vi "DecodeBase64ToImageFile.vi"(8 "error in (no error)":errorcluster, 9 "Base64String":string, 11 "Output FilePath":path) -> (0 "error out":errorcluster, 3 "Output FilePath (FileExtensionAdapted)":path)   [LabVIEW 2020]
doc: "Decode a Base64 Image to a file"
uses:
  <userlib>/_OpenG.lib/file/file.llb/Valid Path - Traditional__ogtk.vi
  <vilib>/Utility/error.llb/Error Cluster From Error Code.vi
  <userlib>/_OpenG.lib/file/file.llb/Convert File Extension (Path)__ogtk.vi
  <vilib>/ErrorRing/Error Ring.xnode
  <userlib>/_OpenG.lib/file/file.llb/openg_file.lvlib
  <vilib>/JDP Science/JDP Science Common Utilities/Base64/Base64 Support.lvlib
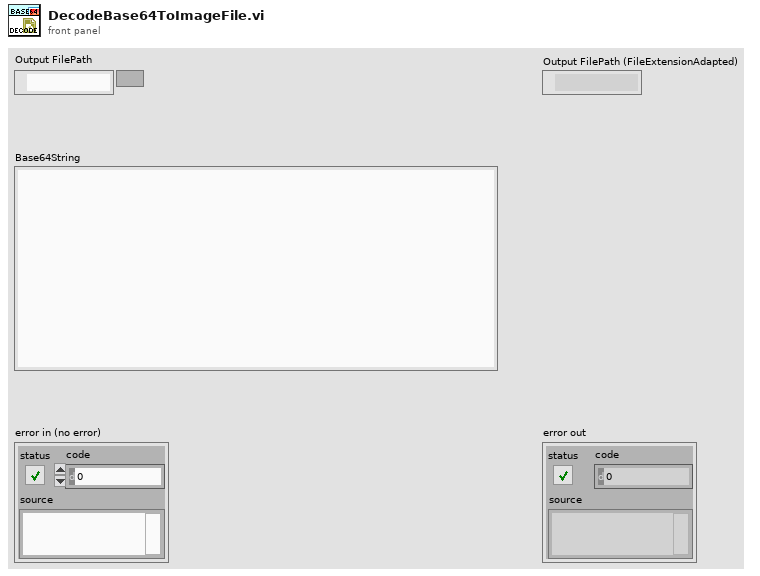
[diagram p1: front panel]
types:
  T1 = enum16{"open", "replace", "create", "open or create", "replace or create", "replace or create with confirmation"}
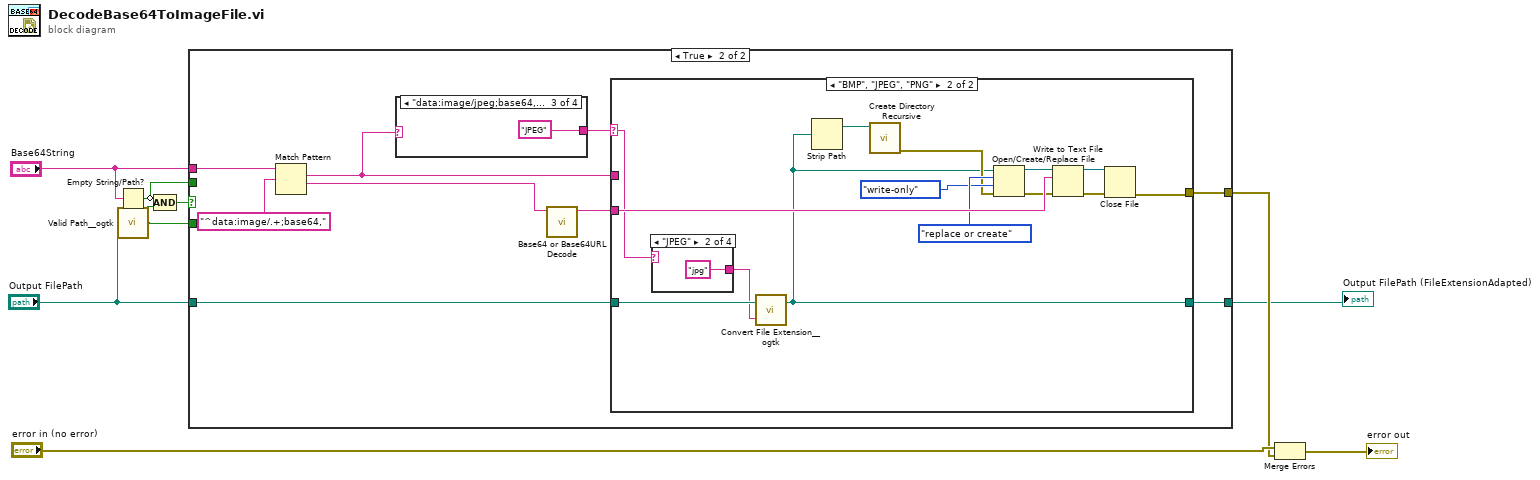
[diagram p0: block diagram]
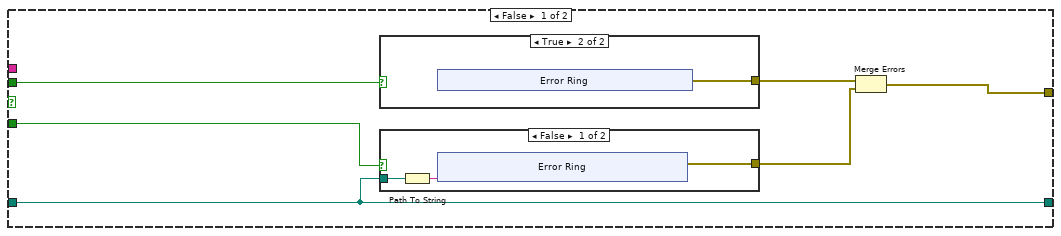
[diagram p2: hidden frame]
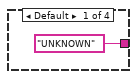
[diagram p5: hidden frame]
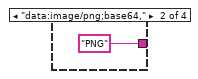
[diagram p6: hidden frame]
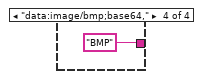
[diagram p7: hidden frame]
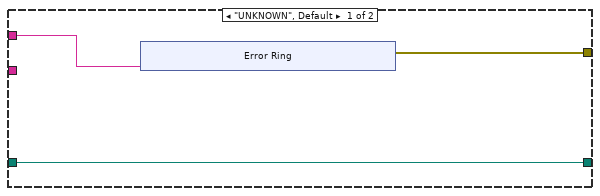
[diagram p8: hidden frame]
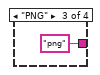
[diagram p10: hidden frame]
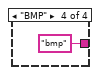
[diagram p11: hidden frame]
diagram:
  n1 = Empty String/Path?(string/path="Base64String") -> (empty?=w2:bool)
  n2 = call-poly <userlib>:"Valid Path__ogtk.vi"("path"="Output FilePath") -> ("valid"=w1:bool)
  n3 = Compound Arithmetic op=AND(invert w2, w1) -> (w3:bool)
  n4 = case shown="True" w3 {
    tunnel: [w12 w40] -> w7
    tunnel: "Base64String" -> [_ w38]
    tunnel: "Output FilePath" -> [w10 w33]
    tunnel: [w10 w32] -> w4
    tunnel: w2 -> [w14 _]
    tunnel: w1 -> [w13 _]
    frame False {
      n5 = case shown="True" w14 {
        tunnel: [_ w26] -> w15
        frame False {
        }
        frame True {
          n6 = xnode "Error Ring"() -> ("error out"=w26:errorcluster)
        }
      }
      n7 = case shown="False" w13 {
        tunnel: [w18 _] -> w11
        tunnel: w10 -> [w16 _]
        frame False {
          n8 = Path To String(path=w16) -> (string=w17:string)
          n9 = xnode "Error Ring"("parameter 0"=w17) -> ("error out"=w18:errorcluster)
        }
        frame True {
        }
      }
      n10 = Merge Errors(w15, w11) -> (w12:errorcluster)
    }
    frame True {
      n11 = Match Pattern(string=w38, regular expression="^data:image/.+;base64,") -> (match substring=w37:string, after substring=w36:string)  [unwired: 1 in, 2 out]
      n12 = case shown="\"data:image/jpeg;base64,\"" w37 {
        tunnel: ["UNKNOWN" "PNG" "JPEG" "BMP"] -> w34
        frame Default {
        }
        frame "data:image/png;base64," {
        }
        frame "data:image/jpeg;base64," {
        }
        frame "data:image/bmp;base64," {
        }
      }
      n13 = call <vilib>:"Base64 or Base64URL Decode.vi"("Base64 or Base64URL"=w36) -> ("Decoded"=w35:string)  [unwired: 10 in]
      n14 = case shown="\"BMP\", \"JPEG\", \"PNG\"" w34 {
        selector: w34 -> [_ w59]
        tunnel: [w47 w61] -> w40
        tunnel: w37 -> [w46 _]
        tunnel: w35 -> [_ w66]
        tunnel: w33 -> [w45 w60]
        tunnel: [w45 w55] -> w32
        frame "UNKNOWN", Default {
          n15 = xnode "Error Ring"("parameter 0"=w46) -> ("error out"=w47:errorcluster)
        }
        frame "BMP", "JPEG", "PNG" {
          n16 = case shown="\"JPEG\"" w59 {
            tunnel: [_ "jpg" "png" "bmp"] -> w58
            frame "UNKNOWN", Default {
            }
            frame "JPEG" {
            }
            frame "PNG" {
            }
            frame "BMP" {
            }
          }
          n17 = call-poly <userlib>:"Convert File Extension__ogtk.vi"("new ending (none)"=w58, "file name"=w60) -> ("new filename"=w55:path)  [unwired: 1 out]
          n18 = Strip Path(path=w55) -> (stripped path=w57:path)  [unwired: 1 out]
          n19 = call <vilib>:"Create Directory Recursive.vi"("directory"=w57) -> ("error out"=w56:errorcluster)  [unwired: 4 in, 2 out]
          n20 = Open/Create/Replace File(file path (use dialog)=w55, error in=w56, operation (0:open)=T1."replace or create", access (0:read/write)=enum16{"read/write", "read-only", "write-only"}."write-only") -> (refnum out=w65:refnum<file>, error out=w63:errorcluster)  [unwired: 2 in, 1 out]
          n21 = Write to Text File(file (use dialog)=w65, text=w66, error in=w63) -> (refnum out=w68:refnum<file>, error out=w67:errorcluster)  [unwired: 1 in, 1 out]
          n22 = Close File(refnum=w68, error in=w67) -> (error out=w61:errorcluster)  [unwired: 1 out]
        }
      }
    }
  }
  "Output FilePath (FileExtensionAdapted)" <- w4
  n23 = Merge Errors("error in (no error)", w7) -> (→"error out":errorcluster)
